vi "module.Layouts.Lite.vi"(7 "DVR":T3, 8 "error in":errorcluster) -> (0 "error out":errorcluster)   [LabVIEW 2020]
uses:
  _controls/element.ctl
  _controls/data.ctl
  camera/camera.lvclass
  _controls/data.ref.ctl
  <vilib>/vision/Image Controls.llb/IMAQ Image.ctl
  _controls/state.ctl
  _controls/data.vars.ctl
  _controls/save_options.ctl
  _controls/flip.ctl
  bus.ctl
  <vilib>/Utility/file.llb/Read Delimited Spreadsheet (I64).vi
panel:
  in  "save":bool
  out "modules":T1[][](array[typedef])
  in  "position":T2(radio)
  in  "clear":bool
  in  "cancel":bool
  in  "Columns":u8=1 min=1 max=10 step=1
  in  "Rows":u8=1 min=1 max=60 step=1
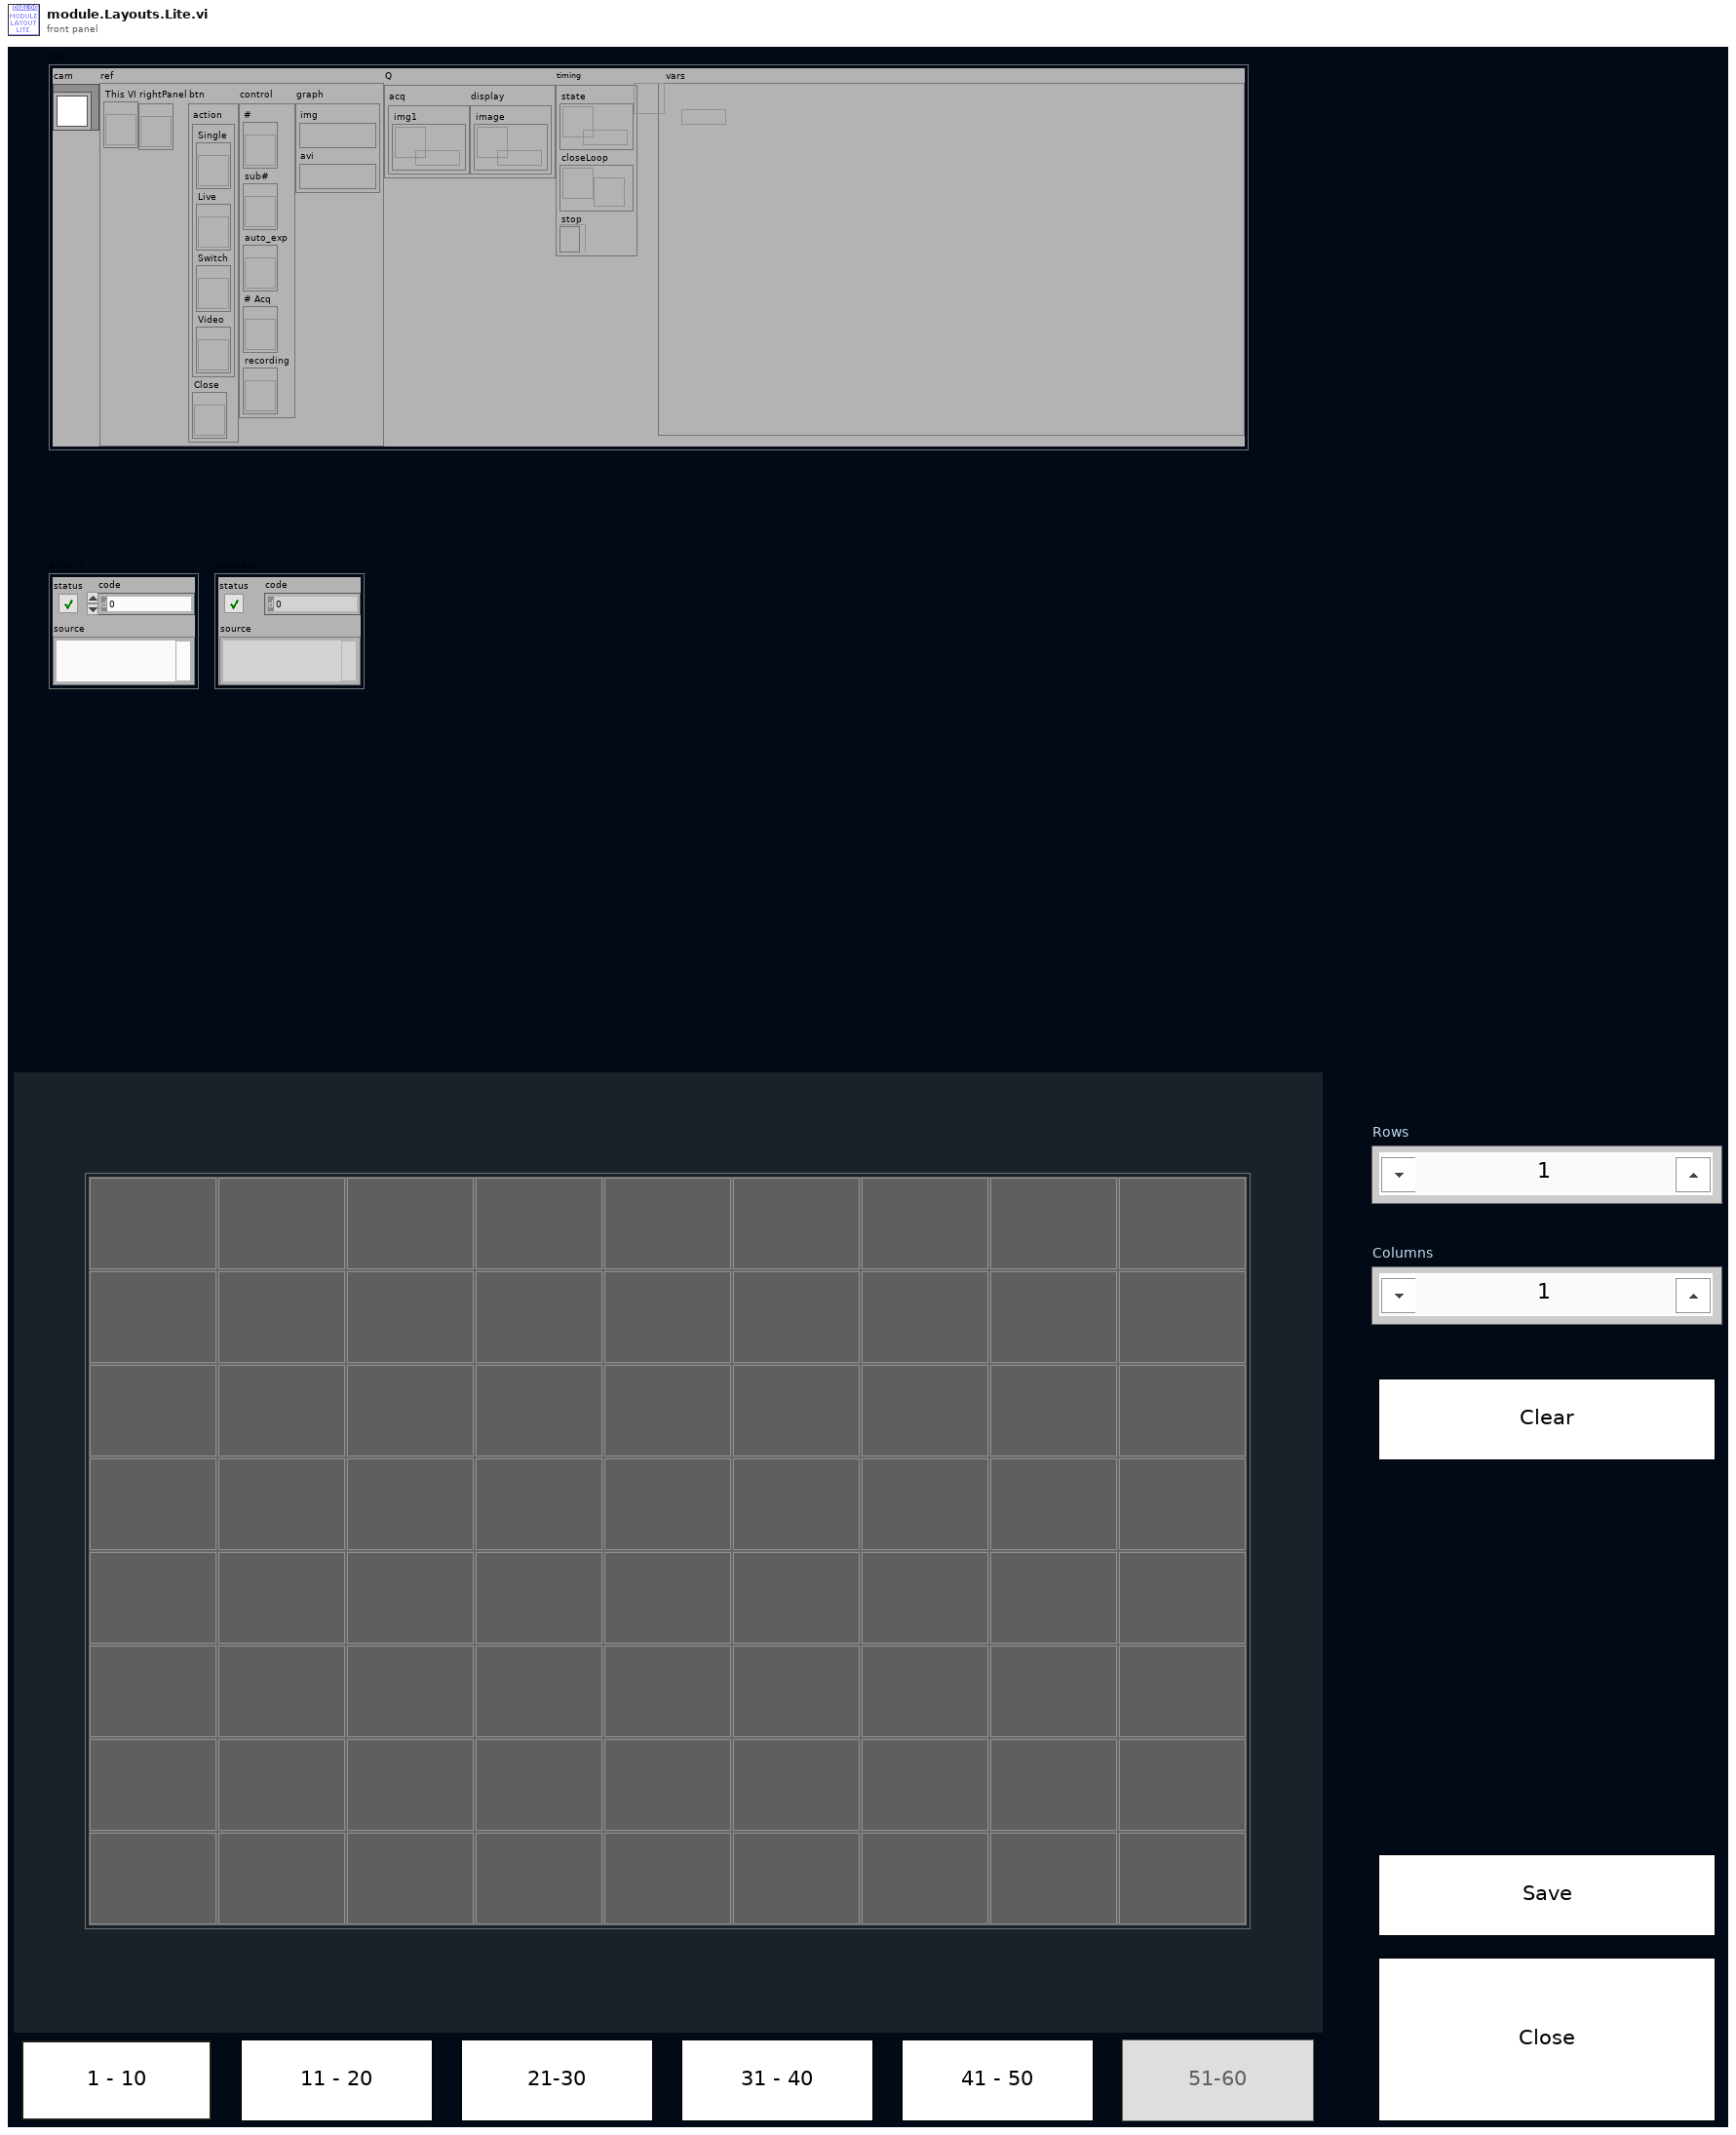
[diagram p1: front panel]
types:
  T1 = typedef "element.ctl" = cluster{"Color Box":u32, "label":string}
  T2 = enum32{"1-10", "11-20", "21-30", "31-40", "41-50", "51-60"}
  T3 = typedef "data.ctl" = cluster{"cam":refnum<class "camera.lvclass">, "ref":T4, "Q":cluster{"acq":cluster{"img1":refnum<queue>}, "display":cluster{"image":refnum<queue>}}, "timing":cluster{"state":refnum<queue>, "closeLoop":refnum<notifier>, "stop":refnum<k4>}, "vars":refnum<data-value>}
  T4 = typedef "data.ref.ctl" = cluster{"This VI":refnum<vi>, "rightPanel":refnum<vi>, "btn":cluster{"action":cluster{"Single":refnum<vi>, "Live":refnum<vi>, "Switch":refnum<vi>, "Video":refnum<vi>}, "Close":refnum<vi>}, "control":cluster{"#":refnum<vi>, "sub#":refnum<vi>, "auto_exp":refnum<vi>, "# Acq":refnum<vi>, "recording":refnum<vi>}, "graph":cluster{"img":T5, "avi":T5}}
  T5 = typedef "IMAQ Image.ctl" = refnum<image>
  T6 = typedef "bus.ctl" = cluster{"ref":cluster{"Columns":refnum<vi>, "rows":refnum<vi>, "position":refnum<vi>, "modules":refnum<vi>, "This VI":refnum<vi>}}
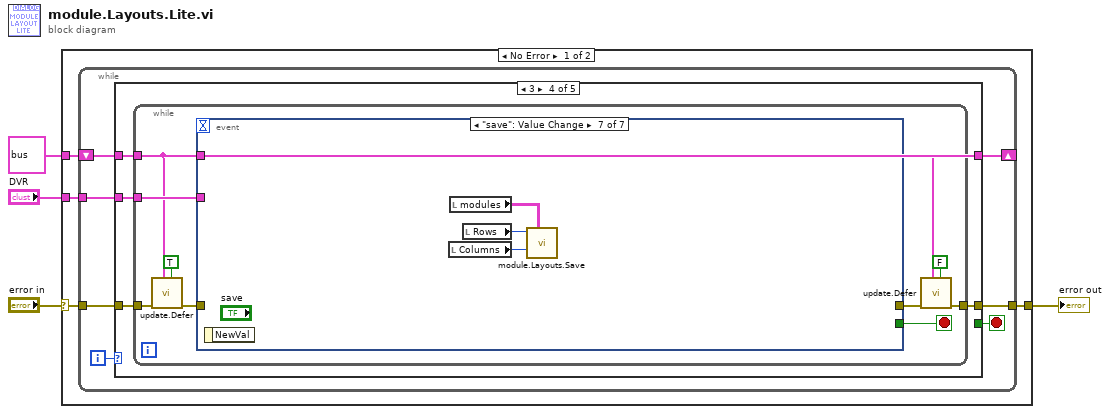
[diagram p0: block diagram]
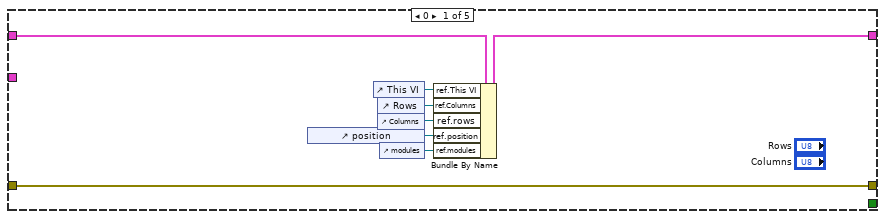
[diagram p2: hidden frame]
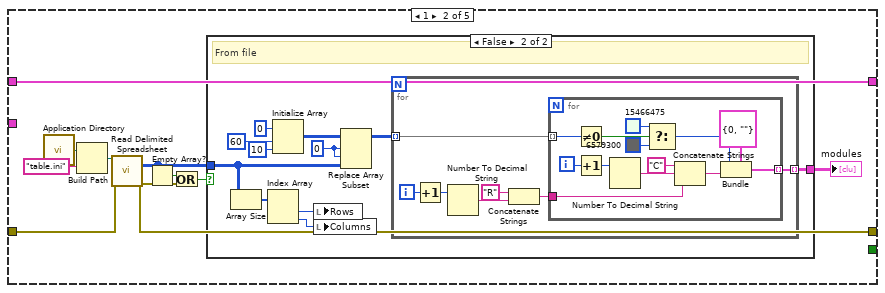
[diagram p3: hidden frame]
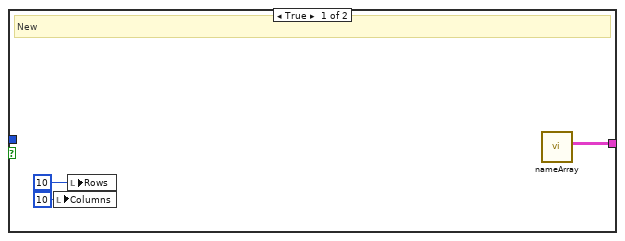
[diagram p4: hidden frame]
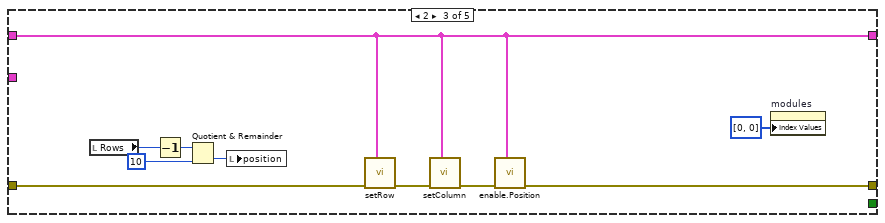
[diagram p5: hidden frame]
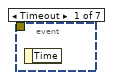
[diagram p6: hidden frame]
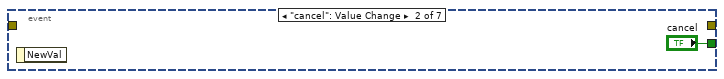
[diagram p7: hidden frame]
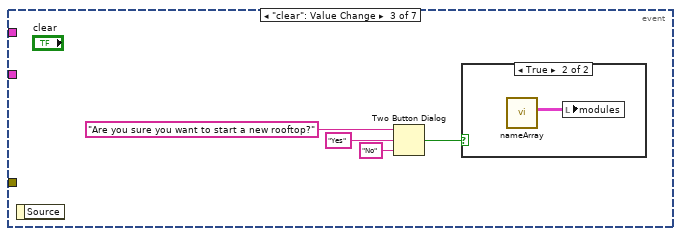
[diagram p8: hidden frame]
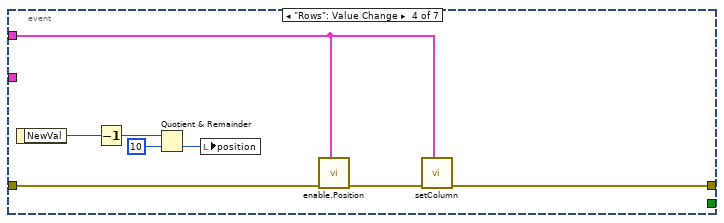
[diagram p10: hidden frame]
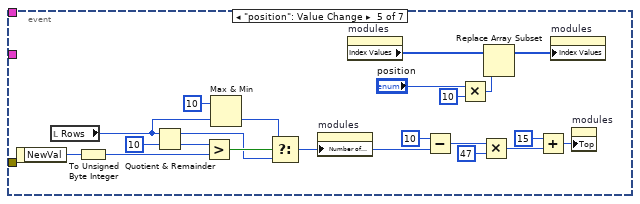
[diagram p11: hidden frame]
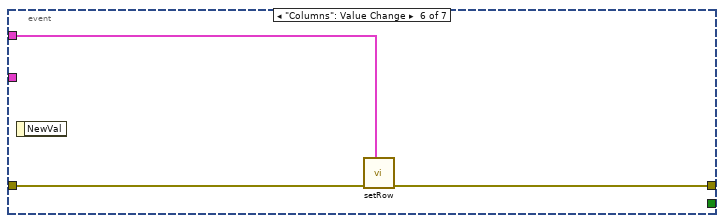
[diagram p12: hidden frame]
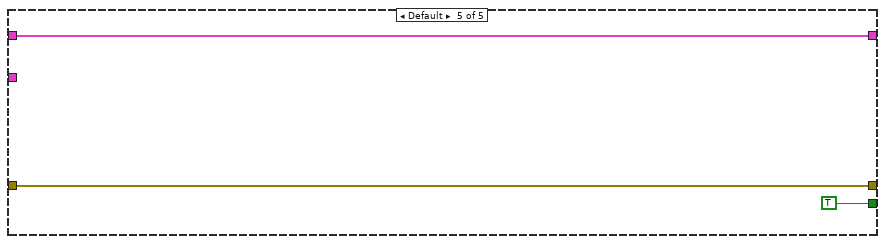
[diagram p13: hidden frame]
diagram:
  n1 = case shown="No Error" "error in" {
    selector: "error in" -> [w6 w135]
    tunnel: [w5 w135] -> w3
    tunnel: "DVR" -> [w8 _]
    tunnel: T6 {"ref"={"Columns"=refnum, "rows"=refnum, "position"=refnum, "modules"=refnum, "This VI"=refnum}} ("bus") -> [w7 _]
    frame No Error {
      n2 = while {
        tunnel: w8 -> [w13]
        shift-right: [w11] -> _
        shift-left: w7 -> [w12]
        tunnel: w6 -> [w10]
        tunnel: [w9] -> w5
        i -> [w15]
        stop <- w14 stop-if-true
        n3 = case shown="3" w15 {
          tunnel: [_ _ _ _ TRUE] -> w14
          tunnel: w13 -> [_ _ _ w81 _]
          tunnel: w12 -> [w23 w26 w73 w78 w133]
          tunnel: [w22 w26 w73 w78 w133] -> w11
          tunnel: w10 -> [w17 w24 w76 w80 w132]
          tunnel: [w17 w25 w72 w79 w132] -> w9
          frame 0 {
            n4 = control-ref of="position"() -> (w21:refnum<vi>)
            n5 = control-ref of="This VI"() -> (w16:refnum<vi>)
            n6 = control-ref of="Rows"() -> (w20:refnum<vi>)
            n7 = control-ref of="Columns"() -> (w19:refnum<vi>)
            n8 = control-ref of="modules"() -> (w18:refnum<vi>)
            n9 = Bundle By Name(cluster=w23, "ref.This VI"=w16, "ref.Columns"=w20, "ref.rows"=w19, "ref.position"=w21, "ref.modules"=w18) -> (w22:T6)
          }
          frame 1 {
            n10 = call <vilib>:"Application Directory.vi"() -> ("Application Directory"=w32:path)
            n11 = Build Path(base path=w32, name or relative path="table.ini" ("format (%d)")) -> (appended path=w30:path)
            n12 = call-poly <vilib>:"Read Delimited Spreadsheet.vi"("file path (dialog if empty)"=w30, "error in (no error)"=w24) -> ("all rows"=w28:i64[][], "error out"=w25:errorcluster)  [unwired: 8 in, 4 out]
            n13 = Empty Array?(array=w28) -> (empty?=w29:bool)
            n14 = Or(x=w29, y=w25) -> (x .or. y?=w27:bool)
            n15 = case shown="False" w27 {
              tunnel: [w34 w47] -> w33
              tunnel: w28 -> [_ w40]
              frame True {
                # "New"
                n16 = local write "Columns"(u8 10 ("Rows")) -> ()
                n17 = local write "Rows"(u8 10 ("Columns")) -> ()
                n18 = call "nameArray.vi"() -> ("Array"=w34:T1[][])  [unwired: 10 in, 1 out]
              }
              frame False {
                w45 = 0 ("index (row)")
                # "From file"
                n19 = Array Size(array=w40) -> (size(s)=w41:i32[])
                n20 = Index Array(array=w41) -> (element #1=w39:i32, element #2=w38:i32)  [unwired: 2 in]
                n21 = Initialize Array(u32 0 ("element"), 60 ("dimension size"), 10 ("dimension size")) -> (w42:u32[][])
                n22 = local write "Rows"(w39) -> ()
                n23 = local write "Columns"(w38) -> ()
                n24 = Replace Array Subset(array=w42, new element=w40, index (row)=w45, index (col)=w45) -> (w44:u32[][])
                n25 = for {
                  tunnel: [w52] -> w47 mode=indexing
                  tunnel: w44 -> [w50] mode=indexing
                  i -> [w54]
                  n26 = Increment(x=w54) -> (x+1=w51:i32)
                  n27 = Number To Decimal String(number=w51) -> (decimal integer string=w53:string)  [unwired: 1 in]
                  n28 = Concatenate Strings("R" ("string"), w53) -> (w49:string)
                  n29 = for {
                    tunnel: w49 -> [w64]
                    tunnel: [w65] -> w52 mode=indexing
                    tunnel: w50 -> [w63] mode=indexing
                    i -> [w57]
                    n30 = Not Equal To 0?(x=w63) -> (x != 0?=w62:bool)
                    n31 = Increment(x=w57) -> (x+1=w55:i32)
                    n32 = Number To Decimal String(number=w55) -> (decimal integer string=w56:string)  [unwired: 1 in]
                    n33 = Select(t=u32 15466475 ("Color Box"), s=w62, f=u32 6579300 ("Color Box")) -> (s? t:f=w60:u32)
                    n34 = Concatenate Strings("C" ("string"), w56, w64) -> (w67:string)
                    n35 = Bundle(cluster=T1 {"Color Box"=0, "label"=""} ("element"), "Color Box"=w60, "label"=w67) -> (w65:T1)
                  }
                }
              }
            }
            "modules" <- w33
          }
          frame 2 {
            n36 = local read "Rows"() -> (w69:u8)
            n37 = Decrement(x=w69) -> (x-1=w68:u8)
            n38 = Quotient & Remainder(x=w68, y=u8 10) -> (floor(x/y)=w70:u8)  [unwired: 1 out]
            n39 = local write "position"(w70) -> ()
            n40 = call "setRow.vi"("bus"=w73, "error in"=w76) -> ("error out"=w75:errorcluster)  [unwired: 9 in]
            n41 = call "setColumn.vi"("bus"=w73, "error in"=w75) -> ("error out"=w74:errorcluster)  [unwired: 9 in]
            n42 = call "enable.Position.vi"("bus"=w73, "error in"=w74) -> ("error out"=w72:errorcluster)  [unwired: 9 in]
            n43 = property on="modules" class="Arr (strict)"("Index Values"=u32[] [0, 0]) -> ()  [unwired: 2 in, 2 out]
          }
          frame 3 {
            n44 = while {
              tunnel: w81 -> [w89]
              tunnel: w80 -> [w86]
              tunnel: [w87] -> w79
              tunnel: w78 -> [w84]
              stop <- w90 stop-if-true
              n45 = call "update.Defer.vi"("Defer Panel Updates"=TRUE, "bus in"=w84, "error in"=w86) -> ("error out"=w85:errorcluster)  [unwired: 8 in]
              n46 = event shown="[6] \"save\": Value Change" {
                selector: _ -> [_ _ _ _ _ _ _]
                dyn-events: _ -> [_ _ _ _ _ _ _]
                timeout: _ -> [_ _ _ _ _ _ _]
                tunnel: [_ "cancel" _ _ _ _ _] -> w90
                tunnel: w89 -> [_ _ _ _ _ _ _]
                tunnel: w85 -> [_ _ _ w97 _ w128 _]
                tunnel: [_ _ _ w103 _ w127 _] -> w88
                tunnel: w84 -> [_ _ _ w104 _ w126 _]
                event Timeout {
                  n47 = event-data() -> ()  [unwired: 1 in, 1 out]
                }
                event "cancel": Value Change {
                  n48 = event-data() -> ()  [unwired: 1 in, 1 out]
                }
                event "clear": Value Change {
                  n49 = event-data() -> ()  [unwired: 1 in, 1 out]
                  n50 = Two Button Dialog(message="Are you sure you want to start a new rooftop?", 1:"No" ("F button name (\"Cancel\")"), 2:"Yes" ("T button name (\"OK\")")) -> (T button?=w92:bool)
                  n51 = case shown="True" w92 {
                    frame False {
                    }
                    frame True {
                      n52 = call "nameArray.vi"() -> ("Array"=w96:T1[][])  [unwired: 10 in, 1 out]
                      n53 = local write "modules"(w96) -> ()
                    }
                  }
                }
                event "Rows": Value Change {
                  n54 = event-data() -> ("NewVal"=w101:u8)  [unwired: 1 in]
                  n55 = Decrement(x=w101) -> (x-1=w100:u8)
                  n56 = Quotient & Remainder(x=w100, y=u8 10) -> (floor(x/y)=w98:u8)  [unwired: 1 out]
                  n57 = local write "position"(w98) -> ()
                  n58 = call "enable.Position.vi"("bus"=w104, "error in"=w97) -> ("error out"=w102:errorcluster)  [unwired: 9 in]
                  n59 = call "setColumn.vi"("bus"=w104, "error in"=w102) -> ("error out"=w103:errorcluster)  [unwired: 9 in]
                }
                event "position": Value Change {
                  n60 = event-data() -> ("NewVal"=w120:T2)  [unwired: 1 in]
                  n61 = local read "Rows"() -> (w115:u8)
                  n62 = To Unsigned Byte Integer(number=w120) -> (unsigned 8bit integer=w118:u8)
                  n63 = Quotient & Remainder(x=w115, y=u8 10 ("x")) -> (x-y*floor(x/y)=w113:u8, floor(x/y)=w117:u8)
                  n64 = Greater?(x=w117, y=w118) -> (0:w116:bool)
                  n65 = Max & Min(x=u8 10, y=w115) -> (min(x,y)=w112:u8)  [unwired: 1 out]
                  n66 = Select(t=w112, s=w116, f=w113) -> (s? t:f=w106:u8)
                  n67 = property on="modules" class="Arr (strict)"("Number of Rows"=w106) -> ()  [unwired: 2 in, 2 out]
                  n68 = property on="modules" class="Arr (strict)"() -> ("Index Values"=w125:u32[])  [unwired: 2 in, 2 out]
                  n69 = Subtract(x=10, y=w106) -> (x-y=w111:i32)
                  n70 = Multiply(x="position", y=10) -> (x*y=w123:u32)
                  n71 = Multiply(x=w111, y=47) -> (x*y=w109:i32)
                  n72 = Replace Array Subset(array=w125, new element=w123) -> (w124:u32[])  [unwired: 1 in]
                  n73 = Add(x=15, y=w109) -> (x+y=w105:i32)
                  n74 = property on="modules" class="Arr (strict)"("Index Values"=w124) -> ()  [unwired: 2 in, 2 out]
                  n75 = property on="modules" class="Arr (strict)"("Top"=w105) -> ()  [unwired: 2 in, 2 out]
                }
                event "Columns": Value Change {
                  n76 = event-data() -> ()  [unwired: 1 in, 1 out]
                  n77 = call "setRow.vi"("bus"=w126, "error in"=w128) -> ("error out"=w127:errorcluster)  [unwired: 9 in]
                }
                event "save": Value Change {
                  n78 = event-data() -> ()  [unwired: 1 in, 1 out]
                  n79 = local read "Columns"() -> (w129:u8)
                  n80 = local read "modules"() -> (w131:T1[][])
                  n81 = local read "Rows"() -> (w130:u8)
                  n82 = call "module.Layouts.Save.vi"("modules"=w131, "Columns"=w129, "Rows"=w130) -> ()  [unwired: 8 in, 1 out]
                }
              }
              n83 = call "update.Defer.vi"("Defer Panel Updates"=FALSE, "bus in"=w84, "error in"=w88) -> ("error out"=w87:errorcluster)  [unwired: 8 in]
            }
          }
          frame Default {
          }
        }
      }
    }
    frame Error {
    }
  }
  "error out" <- w3
